vi "_jkismpp_user_lib_dir.vi"() -> (0 "jkismpp_user.lib_dir":path)   [LabVIEW 2014]
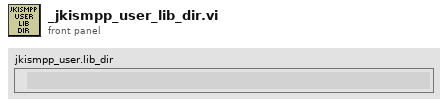
[diagram p1: front panel]
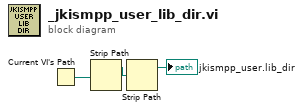
[diagram p0: block diagram]
diagram:
  n1 = Current VI's Path() -> (path=w3:path)
  n2 = Strip Path(path=w3) -> (stripped path=w2:path)  [unwired: 1 out]
  n3 = Strip Path(path=w2) -> (stripped path=→"jkismpp_user.lib_dir":path)  [unwired: 1 out]
